vi "find_max_value_diag.vi"(6 "length":i32, 9 "Frequency array":dbl[](array[numeric]), 10 "Lower Freq":dbl, 11 "Amplitude Array":dbl[](array[numeric])) -> (2 "Frequency":dbl[](array[numeric]), 3 "Peak Amplitude":dbl)   [LabVIEW 2015]
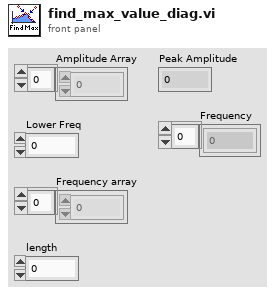
[diagram p1: front panel]
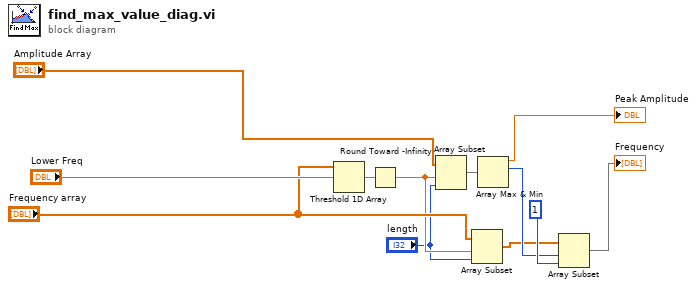
[diagram p0: block diagram]
diagram:
  n1 = Threshold 1D Array(2:"Lower Freq", 3:"Frequency array") -> (0:w7:dbl)  [unwired: 1 in]
  n2 = Round Toward -Infinity(1:w7) -> (0:w4:dbl)
  n3 = Array Subset(array="Amplitude Array", index=w4, length="length") -> (w9:dbl[])
  n4 = Array Subset(array="Frequency array", index=w4, length="length") -> (w2:dbl[])
  n5 = Array Max & Min(array=w9) -> (max value=→"Peak Amplitude":dbl, max index (indices)=w10:i32)  [unwired: 2 out]
  n6 = Array Subset(array=w2, index=w10, length=1) -> (→"Frequency":dbl[])
